vi "AgPSA _Open.vi"(8 "error in (no error)":errorcluster, 9 "External CLK Ref? (True)":bool=TRUE, 10 "Calibrate Now? (True)":bool=TRUE, 11 "PSA In":refnum<visa-resource-name>) -> (0 "error out":errorcluster, 3 "PSA Out":refnum<visa-resource-name>)   [LabVIEW 2015]
uses:
  <instrlib>/Agilent ESA PSA Series/Agilent ESA PSA Series.lvlib
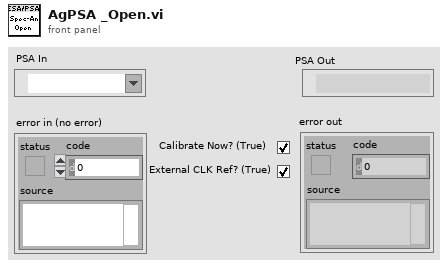
[diagram p1: front panel]
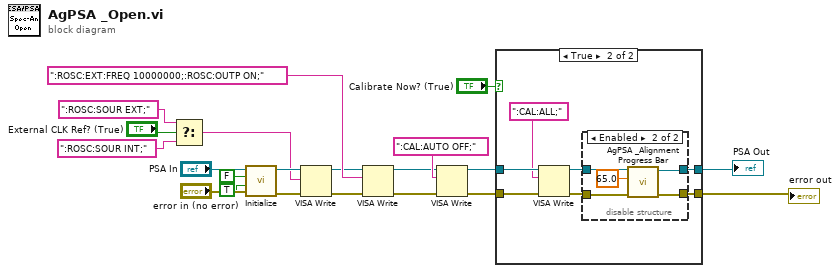
[diagram p0: block diagram]
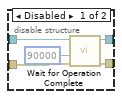
[diagram p3: hidden frame]
diagram:
  n1 = Select(t=":ROSC:SOUR EXT;" ("write buffer"), s="External CLK Ref? (True)", f=":ROSC:SOUR INT;" ("write buffer")) -> (s? t:f=w4:string)
  n2 = call <instrlib>:"Initialize.vi"("error in (no error)"="error in (no error)", "Reset (True)"=TRUE, "ID Query (True)"=FALSE, "VISA resource name"="PSA In") -> ("error out"=w6:errorcluster, "VISA resource name out"=w5:refnum<visa-resource-name>)  [unwired: 6 in]
  n3 = VISA Write(VISA resource name=w5, write buffer=w4, error in (no error)=w6) -> (VISA resource name out=w1:refnum<visa-resource-name>, error out=w2:errorcluster)  [unwired: 1 out]
  n4 = VISA Write(VISA resource name=w1, write buffer=":ROSC:EXT:FREQ 10000000;:ROSC:OUTP ON;", error in (no error)=w2) -> (VISA resource name out=w13:refnum<visa-resource-name>, error out=w12:errorcluster)  [unwired: 1 out]
  n5 = VISA Write(VISA resource name=w13, write buffer=":CAL:AUTO OFF;", error in (no error)=w12) -> (VISA resource name out=w16:refnum<visa-resource-name>, error out=w15:errorcluster)  [unwired: 1 out]
  n6 = case shown="True" "Calibrate Now? (True)" {
    tunnel: [w23 w30] -> w18
    tunnel: [w22 w29] -> w17
    tunnel: w16 -> [w23 w28]
    tunnel: w15 -> [w22 w27]
    frame False {
    }
    frame True {
      n7 = VISA Write(VISA resource name=w28, write buffer=":CAL:ALL;", error in (no error)=w27) -> (VISA resource name out=w26:refnum<visa-resource-name>, error out=w25:errorcluster)  [unwired: 1 out]
      n8 = disable-structure shown="Enabled" {
        disable-tunnel: [w34 w39] -> w30
        disable-tunnel: [w33 w37] -> w29
        disable-tunnel: w26 -> [w32 w40]
        disable-tunnel: w25 -> [w31 w38]
        frame Disabled {
          n9 = call <instrlib>:"Wait for Operation Complete.vi"("error in (no error)"=w31, "Maximum Time (10000ms)"=90000, "VISA resource name"=w32) -> ("error out"=w33:errorcluster, "VISA resource name out"=w34:refnum<visa-resource-name>)  [unwired: 7 in]
        }
        frame Enabled {
          n10 = call "AgPSA _Alignment Progress Bar.vi"("error in (no error)"=w38, "Time Target (s)"=65.0, "VISA resource in"=w40) -> ("error out"=w37:errorcluster, "VISA resource out"=w39:refnum<visa-resource-name>)  [unwired: 6 in, 1 out]
        }
      }
    }
  }
  "PSA Out" <- w18
  "error out" <- w17
